vi "Hybrid car.vi"   [LabVIEW 2016]
uses:
  <vilib>/NXT/Dual Mode Library/Waits/Wait_Num.vi
types:
  T1 = typedef "LVHSConnector.ctl" = refnum<class "BrickReference.lvclass">
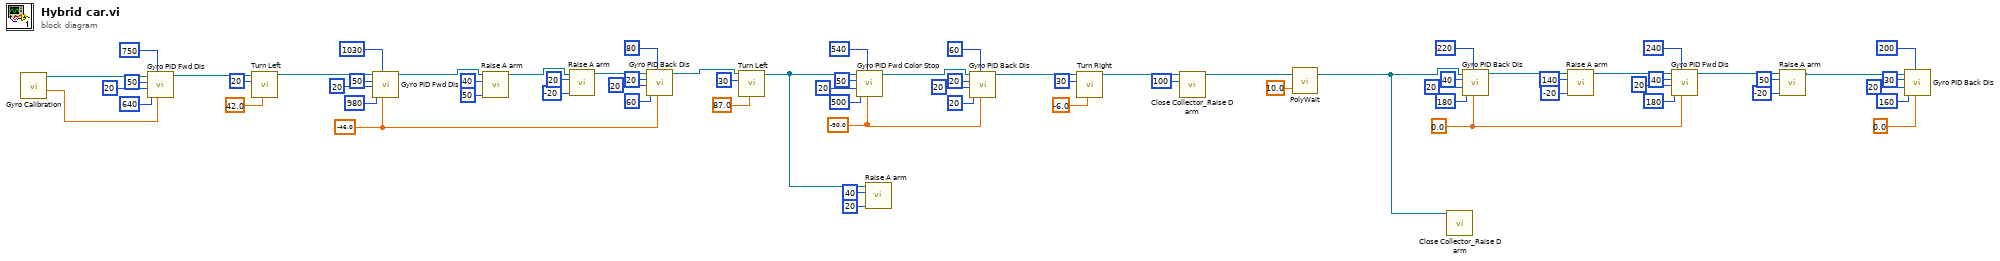
[diagram p0: block diagram]
diagram:
  w33 = sgl 0.0 ("Target angle")
  w28 = sgl -90.0 ("Target angle")
  w6 = sgl -46.0 ("Target angle")
  n1 = call "Gyro Calibration.vi"() -> ("Degrees"=w67:sgl, "NXT/EV3"=w72:T1)  [unwired: 7 in, 1 out]
  n2 = call "Gyro PID Fwd Dis.vi"("Target angle"=w67, "Threshold to stop"=750, "Threshold to slow"=640, "Min. speed"=20, "Max. speed"=50, "EV3 in"=w72) -> ("EV3 out"=w60:T1)  [unwired: 5 in]
  n3 = call "Turn Left.vi"("Turning angle"=sgl 42.0, "Motor B (right)"=i8 20, "EV3 in"=w60) -> ("EV3 out"=w59:T1)  [unwired: 8 in]
  n4 = call "Gyro PID Fwd Dis.vi"("Target angle"=w6, "Threshold to stop"=1030, "Threshold to slow"=980, "Min. speed"=20, "Max. speed"=50, "EV3 in"=w59) -> ("EV3 out"=w16:T1)  [unwired: 5 in]
  n5 = call "Raise A arm.vi"("Power"=i8 50, "Rotation"=40, "EV3 in"=w16) -> ("EV3 out"=w14:T1)  [unwired: 8 in]
  n6 = call "Raise A arm.vi"("Power"=i8 -20, "Rotation"=20, "EV3 in"=w14) -> ("EV3 out"=w12:T1)  [unwired: 8 in]
  n7 = call "Gyro PID Back Dis.vi"("Target angle"=w6, "Threshold to stop"=80, "Threshold to slow"=60, "Min. speed"=20, "Max. speed"=20, "EV3 in"=w12) -> ("EV3 out"=w11:T1)  [unwired: 5 in]
  n8 = call "Turn Left.vi"("Turning angle"=sgl 87.0, "Motor B (right)"=i8 30, "EV3 in"=w11) -> ("EV3 out"=w48:T1)  [unwired: 8 in]
  n9 = call "Gyro PID Fwd Color Stop.vi"("Target angle"=w28, "Threshold to Color"=540, "Threshold to slow"=500, "Min. speed"=20, "Max. speed"=50, "EV3 in"=w48) -> ("EV3 out"=w5:T1)  [unwired: 5 in]
  n10 = call "Raise A arm.vi"("Power"=i8 20, "Rotation"=40, "EV3 in"=w48) -> ()  [unwired: 8 in, 1 out]
  n11 = call "Gyro PID Back Dis.vi"("Target angle"=w28, "Threshold to stop"=60, "Threshold to slow"=20, "Min. speed"=20, "Max. speed"=20, "EV3 in"=w5) -> ("EV3 out"=w27:T1)  [unwired: 5 in]
  n12 = call "Turn Right.vi"("Turning angle"=sgl -6.0, "Motor B (right)"=i8 30, "EV3 in"=w27) -> ("EV3 out"=w4:T1)  [unwired: 8 in]
  n13 = call "Close Collector_Raise D arm.vi"("Rotation"=100, "EV3 in"=w4) -> ("EV3 out"=w2:T1)  [unwired: 9 in]
  n14 = call-poly <vilib>:"PolyWait.vi"("Time (1 sec)"=sgl 10.0, "NXT/EV3"=w2) -> ("NXT/EV3"=w1:T1)  [unwired: 2 in]
  n15 = call "Close Collector_Raise D arm.vi"("EV3 in"=w1) -> ()  [unwired: 10 in, 1 out]
  n16 = call "Gyro PID Back Dis.vi"("Target angle"=w33, "Threshold to stop"=220, "Threshold to slow"=180, "Min. speed"=20, "Max. speed"=40, "EV3 in"=w1) -> ("EV3 out"=w39:T1)  [unwired: 5 in]
  n17 = call "Raise A arm.vi"("Power"=i8 -20, "Rotation"=140, "EV3 in"=w39) -> ("EV3 out"=w38:T1)  [unwired: 8 in]
  n18 = call "Gyro PID Fwd Dis.vi"("Target angle"=w33, "Threshold to stop"=240, "Threshold to slow"=180, "Min. speed"=20, "Max. speed"=40, "EV3 in"=w38) -> ("EV3 out"=w24:T1)  [unwired: 5 in]
  n19 = call "Raise A arm.vi"("Power"=i8 -20, "Rotation"=50, "EV3 in"=w24) -> ("EV3 out"=w18:T1)  [unwired: 8 in]
  n20 = call "Gyro PID Back Dis.vi"("Target angle"=sgl 0.0, "Threshold to stop"=200, "Threshold to slow"=160, "Min. speed"=20, "Max. speed"=30, "EV3 in"=w18) -> ()  [unwired: 5 in, 1 out]
